vi "Start.vi"(8 "error in (no error)":errorcluster, 11 "Tovey9150 in":refnum<class "Tovey 9150.lvclass">) -> (0 "error out":errorcluster, 3 "Tovey9150 out":refnum<class "Tovey 9150.lvclass">)   [LabVIEW 2015, in "Tovey 9150.lvclass"]
uses:
  Tovey 9150.lvclass
  Tovey 9150.lvclass/Tovey 9150.ctl
  Common_SerialProtocols/SerialCommunicator/SerialCommunicator.lvclass
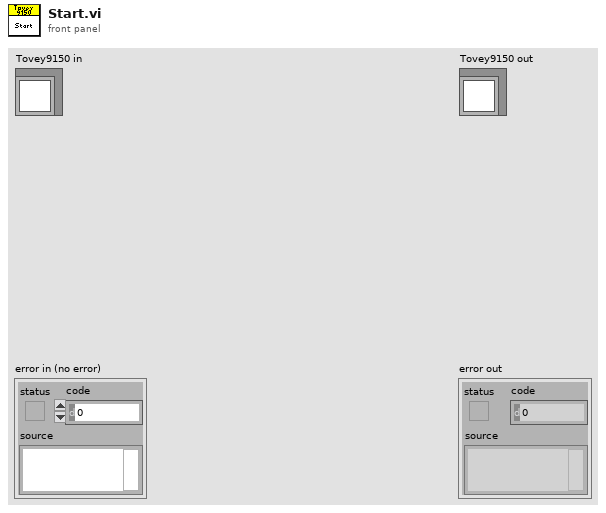
[diagram p1: front panel]
types:
  T1 = typedef "SerialProtocols.lvlib/SerialConfig.ctl" = cluster{"Serial Protocol":T2, "Protocol Parameters":T3, "Serial Message Parameters":T4}
  T2 = typedef "SerialProtocols.lvlib/SerialProtocol.ctl" = enum16{"RS232", "RS485", "SerialSimulator"}
  T3 = typedef "SerialProtocols.lvlib/ProtocolParameters.ctl" = cluster{"VISA resource name":refnum<visa-resource-name>, "Baud Rate":u32, "Data Bits":u16, "Parity":enum16{"None", "Odd", "Even", "Mark", "Space"}, "Flow Control":u16, "Stop Bits":u16, "Timeout (ms)":u32}
  T4 = typedef "SerialProtocols.lvlib/SerialMessageParameters.ctl" = cluster{"Byte Count":u32, "Enable Termination Character":bool, "Termination Char":u8}
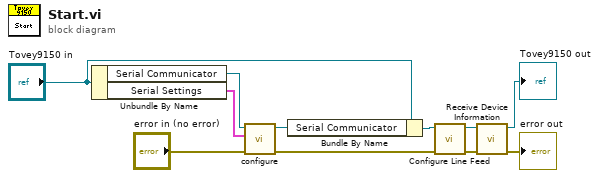
[diagram p0: block diagram]
diagram:
  n1 = Unbundle By Name("Tovey9150 in") -> ("Serial Communicator"=w11:refnum<class "SerialCommunicator.lvclass">, "Serial Settings"=w10:T1)
  n2 = call-dynamic "configure.vi"("error in (no error)"="error in (no error)", "SerialConfig"=w10, "SerialCommunicator in"=w11) -> ("error out"=w3:errorcluster, "SerialCommunicator out"=w9:refnum<class "SerialCommunicator.lvclass">)  [unwired: 7 in]
  n3 = Bundle By Name(cluster="Tovey9150 in", "Serial Communicator"=w9) -> (w7:refnum<class "Tovey 9150.lvclass">)
  n4 = call "Configure Line Feed.vi"("error in (no error)"=w3, "Tovey9150 in"=w7) -> ("error out"=w2:errorcluster, "Tovey9150 out"=w6:refnum<class "Tovey 9150.lvclass">)  [unwired: 8 in]
  n5 = call "Receive Device Information.vi"("error in (no error)"=w2, "Tovey9150 in"=w6) -> ("error out"=→"error out":errorcluster, "Tovey9150 out"=→"Tovey9150 out":refnum<class "Tovey 9150.lvclass">)  [unwired: 8 in]
